vi "Update Values.vi"(4 "MXN?":bool, 5 "Soda?":bool, 6 "Index":i32, 7 "Inventario":dbl, 8 "error in (no error)":errorcluster, 9 "Costo":dbl, 10 "Producto":string, 11 "UI Actor in":refnum<class "UI Actor.lvclass">) -> (0 "error out":errorcluster, 3 "UI Actor out":refnum<class "UI Actor.lvclass">)   [LabVIEW 2020, in "UI Actor.lvlib" / "UI Actor.lvclass"]
uses:
  UI Actor.lvclass
  C:/Program Files (x86)/National Instruments/LabVIEW 2020/vi.lib/ActorFramework/Actor/Actor.lvclass
  UI Actor.lvclass/UI Actor.ctl
  Nestle Actor Messages/Update inventary Msg/Update inventary Msg.lvclass/Update inventary Msg.ctl
  <vilib>/ActorFramework/Message Enqueuer/Message Enqueuer.lvclass/Message Enqueuer.ctl
  Soda Actor Messages/Update Inventary Msg/Update Inventary Msg.lvclass/Update Inventary Msg.ctl
  <vilib>/ActorFramework/Actor/Actor.lvclass/Actor.ctl
  USD Actor Messages/Update Coins Msg/Update Coins Msg.lvclass/Update Coins Msg.ctl
  MXN Actor Messages/Update Coins Msg/Update Coins Msg.lvclass/Update Coins Msg.ctl
  UI Actor Messages/creditUpdate Msg/creditUpdate Msg.lvclass/creditUpdate Msg.ctl
  MSG Messages/Update MSG Msg/Update MSG Msg.lvclass/Update MSG Msg.ctl
  <vilib>/ActorFramework/Message Enqueuer/Enqueue.vi
  Nestle Actor Messages/Update inventary Msg/Update inventary Msg.lvclass
  C:/Program Files (x86)/National Instruments/LabVIEW 2020/vi.lib/ActorFramework/Message/Message.lvclass
  Soda Actor Messages/Update Inventary Msg/Update Inventary Msg.lvclass
  USD Actor Messages/Update Coins Msg/Update Coins Msg.lvclass
  MXN Actor Messages/Update Coins Msg/Update Coins Msg.lvclass
  UI Actor Messages/creditUpdate Msg/creditUpdate Msg.lvclass
  MSG Messages/Update MSG Msg/Update MSG Msg.lvclass
  <vilib>/ActorFramework/Message Priority Queue/Priority Enqueue.vi
  <vilib>/ActorFramework/Actor/Actor.lvclass
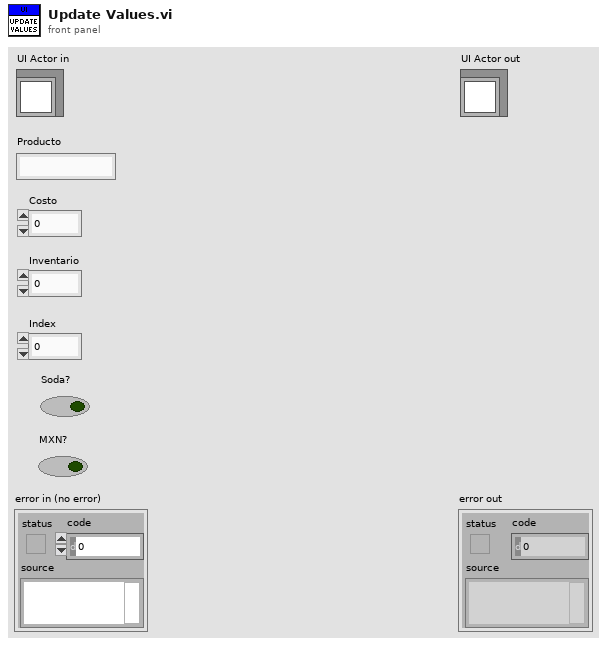
[diagram p1: front panel]
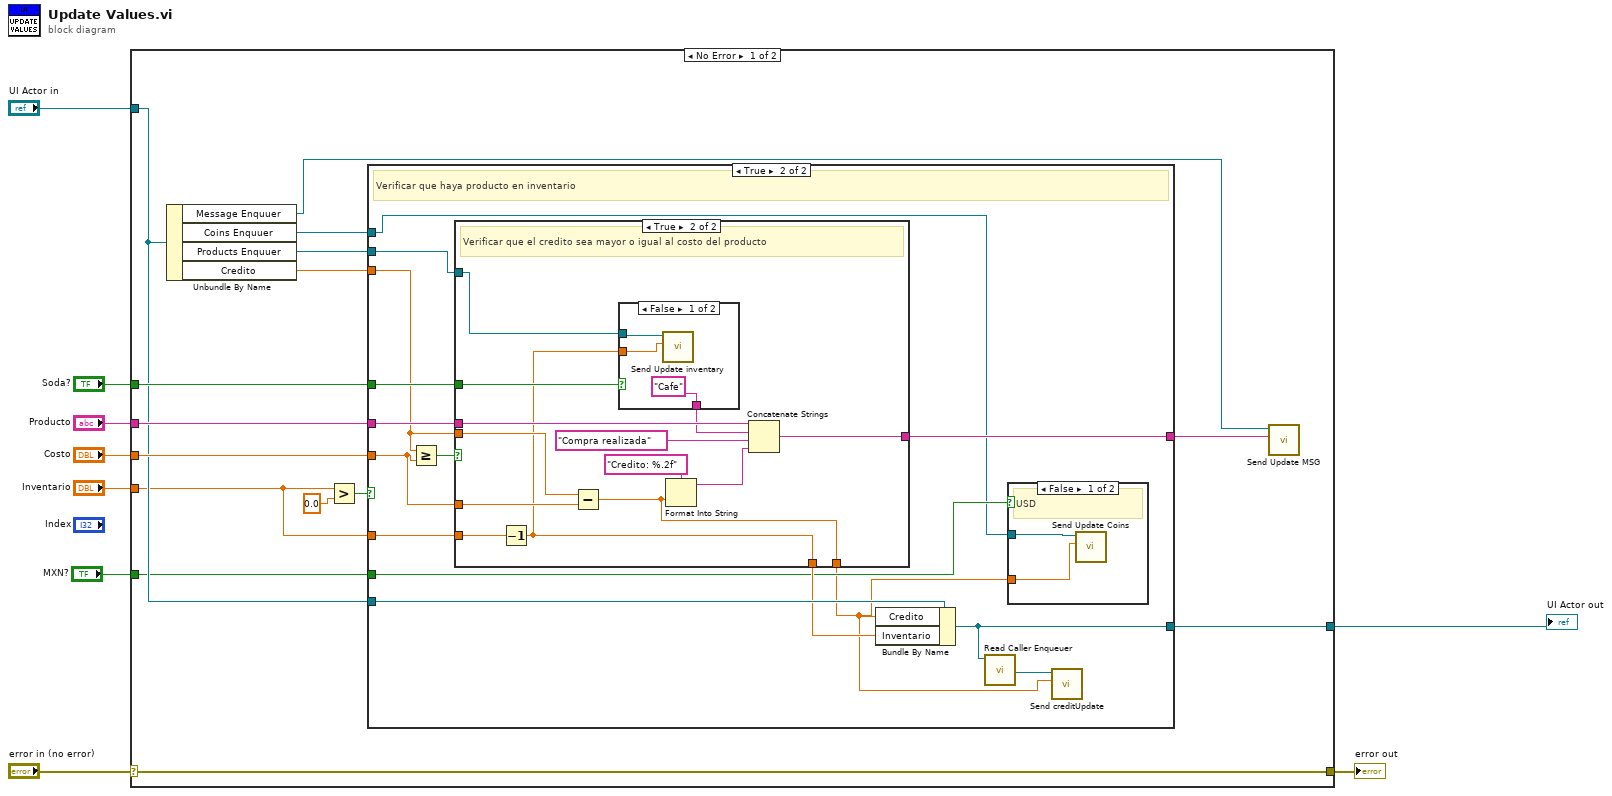
[diagram p0: block diagram]
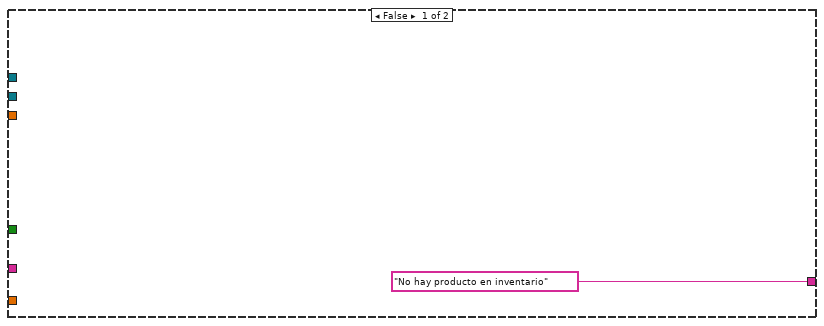
[diagram p2: hidden frame]
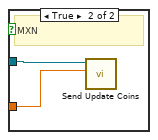
[diagram p3: hidden frame]
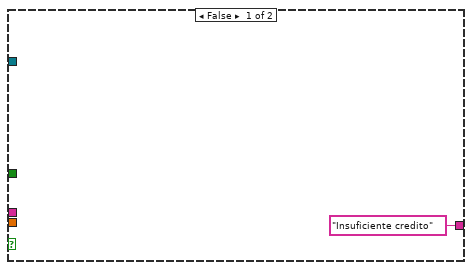
[diagram p4: hidden frame]
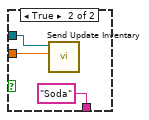
[diagram p5: hidden frame]
diagram:
  n1 = case shown="No Error" "error in (no error)" {
    selector: "error in (no error)" -> [w18 w66]
    tunnel: [w18 w66] -> w8
    tunnel: [w14 w65] -> w6
    tunnel: "UI Actor in" -> [w15 w65]
    tunnel: "Producto" -> [w24 _]
    tunnel: "Soda?" -> [w23 _]
    tunnel: "Costo" -> [w21 _]
    tunnel: "Inventario" -> [w13 _]
    tunnel: "MXN?" -> [w11 _]
    frame No Error {
      n2 = Unbundle By Name(w15) -> ("Message Enquuer"=w19:refnum<class "Message Enqueuer.lvclass">, "Coins Enquuer"=w10:refnum<class "Message Enqueuer.lvclass">, "Products Enquuer"=w12:refnum<class "Message Enqueuer.lvclass">, "Credito"=w22:dbl)
      n3 = Greater?(x=w13, y=0.0) -> (0:w17:bool)
      n4 = case shown="True" w17 {
        tunnel: w24 -> [_ w40]
        tunnel: w23 -> [_ w39]
        tunnel: w22 -> [_ w37]
        tunnel: w21 -> [_ w36]
        tunnel: ["No hay producto en inventario" w35] -> w20
        tunnel: w15 -> [_ w34]
        tunnel: [_ w33] -> w14
        tunnel: w13 -> [_ w32]
        tunnel: w12 -> [_ w31]
        tunnel: w11 -> [_ w28]
        tunnel: w10 -> [_ w27]
        frame False {
        }
        frame True {
          # "Verificar que haya producto en inventario"
          n5 = Greater Or Equal?(x=w37, y=w36) -> (x >= y?=w38:bool)
          n6 = case shown="True" w38 {
            tunnel: w40 -> [_ w58]
            tunnel: w39 -> [_ w56]
            tunnel: w37 -> [_ w52]
            tunnel: w36 -> [_ w51]
            tunnel: ["Insuficiente credito" w50] -> w35
            tunnel: w32 -> [_ w49]
            tunnel: w31 -> [_ w48]
            tunnel: [_ w47] -> w30
            tunnel: [_ w46] -> w26
            frame False {
            }
            frame True {
              # "Verificar que el credito sea mayor o igual al costo del producto"
              n7 = Decrement(x=w49) -> (x-1=w47:dbl)
              n8 = Subtract(x=w52, y=w51) -> (x-y=w46:dbl)
              n9 = case shown="False" w56 {
                tunnel: ["Cafe" ("string") "Soda" ("string")] -> w57
                tunnel: w47 -> [w59 w63]
                tunnel: w48 -> [w60 w62]
                frame False {
                  n10 = call "Send Update inventary.vi"("Inventario"=w59, "Message Enqueuer"=w60) -> ()  [unwired: 8 in, 2 out]
                }
                frame True {
                  n11 = call "Send Update Inventary.vi"("Inventario"=w63, "Message Enqueuer"=w62) -> ()  [unwired: 8 in, 2 out]
                }
              }
              n12 = Format Into String(format string="Credito: %.2f", w46) -> (resulting string=w54:string)  [unwired: 2 in, 1 out]
              n13 = Concatenate Strings(w58, w57, "Compra realizada" ("string"), w54) -> (w50:string)
            }
          }
          n14 = Bundle By Name(cluster=w34, "Credito"=w26, "Inventario"=w30) -> (w33:refnum<class "UI Actor.lvclass">)
          n15 = call <vilib>:"Read Caller Enqueuer.vi"("Actor"=w33) -> ("Caller Enqueuer"=w29:refnum<class "Message Enqueuer.lvclass">)  [unwired: 10 in]
          n16 = case shown="False" w28 {
            tunnel: w27 -> [w42 w44]
            tunnel: w26 -> [w41 w43]
            frame False {
              # "USD"
              n17 = call "Send Update Coins.vi"("Credito Update"=w41, "Message Enqueuer"=w42) -> ()  [unwired: 8 in, 2 out]
            }
            frame True {
              # "MXN"
              n18 = call "Send Update Coins.vi"("Credito Update"=w43, "Message Enqueuer"=w44) -> ()  [unwired: 8 in, 2 out]
            }
          }
          n19 = call "Send creditUpdate.vi"("Credit"=w26, "Message Enqueuer"=w29) -> ()  [unwired: 8 in, 2 out]
        }
      }
      n20 = call "Send Update MSG.vi"("Update message"=w20, "Message Enqueuer"=w19) -> ()  [unwired: 8 in, 2 out]
    }
    frame Error {
    }
  }
  "error out" <- w8
  "UI Actor out" <- w6
